vi "Initialise.vi"(4 "Rate (Hz)":dbl, 6 "Initial DI":T1, 8 "error in (no error)":errorcluster, 9 "Robot Frame":string, 10 "Robot Name":string, 11 "Master in":refnum<class "GripsMaster.lvclass">) -> (0 "error out":errorcluster, 3 "Master out":refnum<class "GripsMaster.lvclass">)   [LabVIEW 2013, in "GripsMaster.lvclass"]
uses:
  GripsMaster.lvclass
  controls/Digital Values.ctl
  controls/Analog Values.ctl
  GripsMaster.lvclass/GripsMaster.ctl
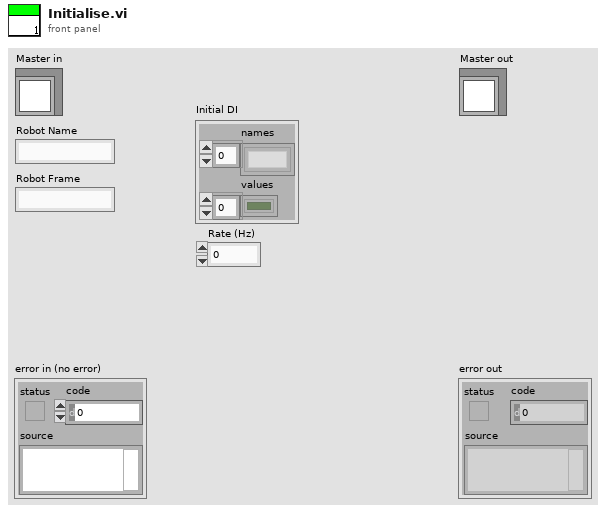
[diagram p1: front panel]
types:
  T1 = typedef "Digital Values.ctl" = cluster{"names":string[], "values":bool[]}
  T2 = typedef "Analog Values.ctl" = cluster{"names":string[], "values":dbl[]}
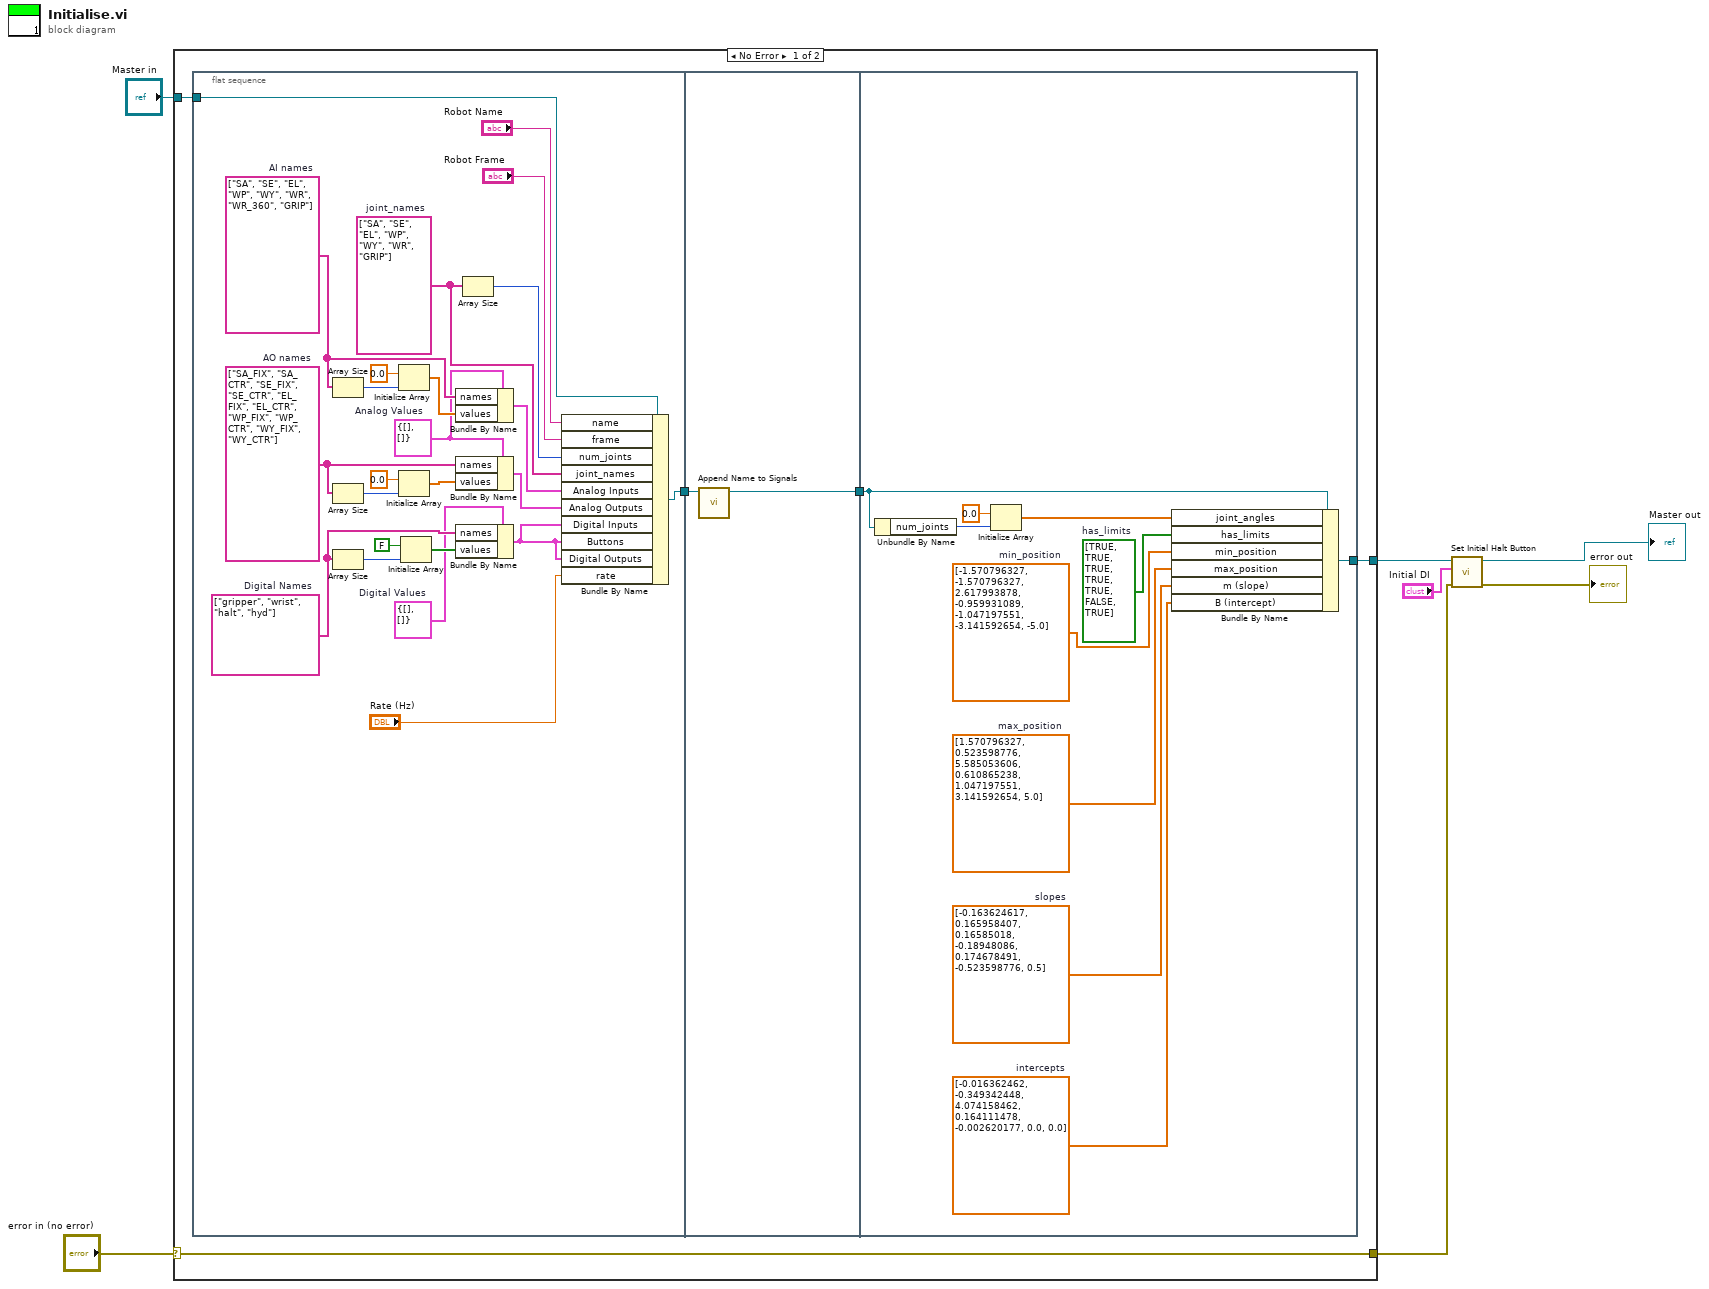
[diagram p0: block diagram]
diagram:
  n1 = case shown="No Error" "error in (no error)" {
    selector: "error in (no error)" -> [w8 w50]
    tunnel: [w8 w50] -> w4
    tunnel: [w10 w49] -> w5
    tunnel: "Master in" -> [w12 w49]
    frame No Error {
      n2 = flat-sequence {
        tunnel: w12 -> [w36]
        tunnel: [w17] -> w11
        tunnel: w11 -> [w38]
        tunnel: [w37] -> w9
        tunnel: [w48] -> w10
        tunnel: w9 -> [w42]
        frame #0 {
          w24 = T2 {"names"=[], "values"=[]}  # Analog Values
          w21 = string[] ["gripper", "wrist", "halt", "hyd"]  # Digital Names
          w32 = string[] ["SA_FIX", "SA_CTR", "SE_FIX", "SE_CTR", "EL_FIX", "EL_CTR", "WP_FIX", "WP_CTR", "WY_FIX", "WY_CTR"]  # AO names
          w29 = string[] ["SA", "SE", "EL", "WP", "WY", "WR", "WR_360", "GRIP"]  # AI names
          w15 = T1 {"names"=[], "values"=[]}  # Digital Values
          w19 = string[] ["SA", "SE", "EL", "WP", "WY", "WR", "GRIP"]  # joint_names
          n3 = Array Size(array=w29) -> (size(s)=w28:i32)
          n4 = Array Size(array=w32) -> (size(s)=w31:i32)
          n5 = Array Size(array=w21) -> (size(s)=w22:i32)
          n6 = Initialize Array(0.0 ("element"), w28) -> (w26:dbl[])
          n7 = Initialize Array(0.0 ("element"), w31) -> (w30:dbl[])
          n8 = Initialize Array(FALSE, w22) -> (w16:bool[])
          n9 = Bundle By Name(cluster=w24, "names"=w29, "values"=w26) -> (w25:T2)
          n10 = Bundle By Name(cluster=w24, "names"=w32, "values"=w30) -> (w23:T2)
          n11 = Bundle By Name(cluster=w15, "names"=w21, "values"=w16) -> (w14:T1)
          n12 = Array Size(array=w19) -> (size(s)=w18:i32)
          n13 = Bundle By Name(cluster=w36, "name"="Robot Name", "frame"="Robot Frame", "num_joints"=w18, "joint_names"=w19, "Analog Inputs"=w25, "Analog Outputs"=w23, "Digital Inputs"=w14, "Buttons"=w14, "Digital Outputs"=w14, "rate"="Rate (Hz)") -> (w17:refnum<class "GripsMaster.lvclass">)
        }
        frame #1 {
          n14 = call "Append Name to Signals.vi"("GripsMaster in"=w38) -> ("GripsMaster out"=w37:refnum<class "GripsMaster.lvclass">)  [unwired: 9 in, 1 out]
        }
        frame #2 {
          w43 = dbl[] [-0.016362462, -0.349342448, 4.074158462, 0.164111478, -0.002620177, 0.0, 0.0]  # intercepts
          w44 = dbl[] [-0.163624617, 0.165958407, 0.16585018, -0.18948086, 0.174678491, -0.523598776, 0.5]  # slopes
          w45 = dbl[] [-1.570796327, -1.570796327, 2.617993878, -0.959931089, -1.047197551, -3.141592654, -5.0]  # min_position
          w46 = dbl[] [1.570796327, 0.523598776, 5.585053606, 0.610865238, 1.047197551, 3.141592654, 5.0]  # max_position
          w47 = bool[] [TRUE, TRUE, TRUE, TRUE, TRUE, FALSE, TRUE]  # has_limits
          n15 = Unbundle By Name(w42) -> ("num_joints"=w40:i32)
          n16 = Initialize Array(0.0 ("element"), w40) -> (w39:dbl[])
          n17 = Bundle By Name(cluster=w42, "joint_angles"=w39, "has_limits"=w47, "min_position"=w45, "max_position"=w46, "m (slope)"=w44, "B (intercept)"=w43) -> (w48:refnum<class "GripsMaster.lvclass">)
        }
      }
    }
    frame Error {
    }
  }
  n18 = call "Set Initial Halt Button.vi"("error in (no error)"=w4, "Digital Inputs"="Initial DI", "GripsMaster in"=w5) -> ("error out"=→"error out":errorcluster, "GripsMaster out"=→"Master out":refnum<class "GripsMaster.lvclass">)  [unwired: 7 in]
